vi "SS2 Live_Next Image Acquisition Step.vi"(8 "Error In":errorcluster, 9 "Message in":string, 11 "SS2 Live Internal Variables in":T3={"okCFrontPanelDevices Refnum"=refnum, "Device Refnum"=refnum, "Display Image"=refnum, "# Live Images"=0, "relative s"=0.0, "# Image Sets"=0, "Message"="", "Current Image Set"=0, "# Datasets"=0, "Current Dataset"=0, "Live Mode"=FALSE, "Recording Mode"=FALSE, "Record Button"=refnum, "Live Button"=refnum, "SS2 Live Gate Data Q Name"="SS2 Live Gate Data Q", "Discard First Image"=FALSE, "Image Information"={"Save ROI Only"=FALSE, "Left"=0, "Top"=0, "Right"=0, "Bottom"=0, "Use Current ROI"=FALSE}, "Image Binning Options"={"Use Image Binning"=FALSE, "X Bin"=1, "Y Bin"=1}} {"Image Binning Options"."Y Bin" min=1; "Image Binning Options"."X Bin" min=1}) -> (0 "Error Out":errorcluster, 1 "Message out":string, 2 "SS2 Live Atomic Action":T1={"SS2 Q Event"=enum."Idle", "Data"=variant}, 3 "SS2 Live Internal Variables out":T3={"okCFrontPanelDevices Refnum"=refnum, "Device Refnum"=refnum, "Display Image"=refnum, "# Live Images"=0, "relative s"=0.0, "# Image Sets"=0, "Message"="", "Current Image Set"=0, "# Datasets"=0, "Current Dataset"=0, "Live Mode"=FALSE, "Recording Mode"=FALSE, "Record Button"=refnum, "Live Button"=refnum, "SS2 Live Gate Data Q Name"="SS2 Live Gate Data Q", "Discard First Image"=FALSE, "Image Information"={"Save ROI Only"=FALSE, "Left"=0, "Top"=0, "Right"=0, "Bottom"=0, "Use Current ROI"=FALSE}, "Image Binning Options"={"Use Image Binning"=FALSE, "X Bin"=1, "Y Bin"=1}} {"Image Binning Options"."Y Bin" min=1; "Image Binning Options"."X Bin" min=1})   [LabVIEW 2019]
uses:
  SS2 Live Internal Variables.ctl
  C:/UCLA Thinkpad Google Drive/LabVIEW 2019 SP1/builds/SS2 Live Distribution/Opal Kelly/C# Wrapper/libFrontPanel-csharp.dll
  Opal Kelly/C# Wrapper/libFrontPanel-csharp.dll
  <vilib>/vision/Image Controls.llb/IMAQ Image.ctl
  SS2 Live_Image ROI Information.ctl
  Phasor/Image Binning Options.ctl
  SS2 Q [Element].ctl
  SS2 Q Event List.ctl
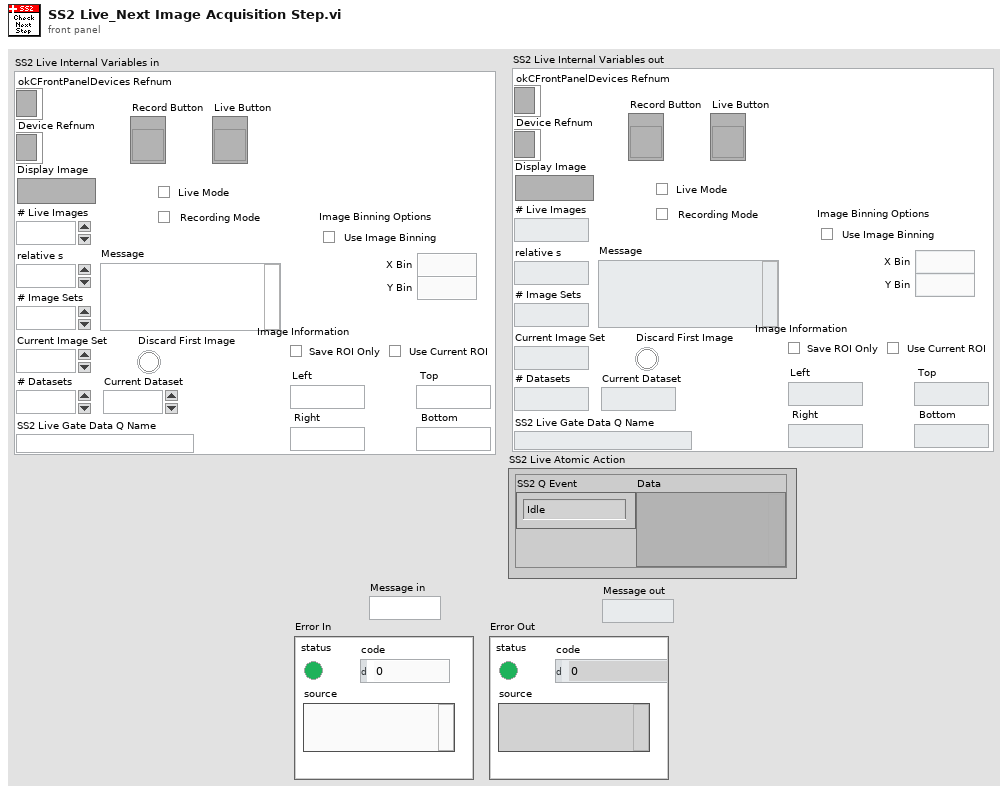
[diagram p1: front panel]
types:
  T1 = typedef "SS2 Q [Element].ctl" = cluster{"SS2 Q Event":T2, "Data":variant}
  T2 = typedef "SS2 Q Event List.ctl" = enum16{"---- UI ----", "Idle", "Initialization", "Quit", "---- DAQ ----", "Start Recording", "Start Live Acquisition", "Initialize Recording Mode", "Initialize FPGA (Live Mode)", "Get Image Set", "Get Single Image", "Update Image Display", "Stop Live Acquisition", "Stop Data Recording", "---- Image ----", "Copy Data to Clipboard", "Set Image Palette", "Save Displayed Image with Overlay", "Save Image Data as TIFF"}
  T3 = typedef "SS2 Live Internal Variables.ctl" = cluster{"okCFrontPanelDevices Refnum":refnum<k24>, "Device Refnum":refnum<k24>, "Display Image":T4, "# Live Images":i32, "relative s":dbl, "# Image Sets":i32, "Message":string, "Current Image Set":i32, "# Datasets":i32, "Current Dataset":i32, "Live Mode":bool, "Recording Mode":bool, "Record Button":refnum<vi>, "Live Button":refnum<vi>, "SS2 Live Gate Data Q Name":string, "Discard First Image":bool, "Image Information":T5, "Image Binning Options":T6}
  T4 = typedef "IMAQ Image.ctl" = refnum<image>
  T5 = typedef "SS2 Live_Image ROI Information.ctl" = cluster{"Save ROI Only":bool, "Left":u16, "Top":u16, "Right":u16, "Bottom":u16, "Use Current ROI":bool}
  T6 = typedef "Image Binning Options.ctl" = cluster{"Use Image Binning":bool, "X Bin":i32, "Y Bin":i32}
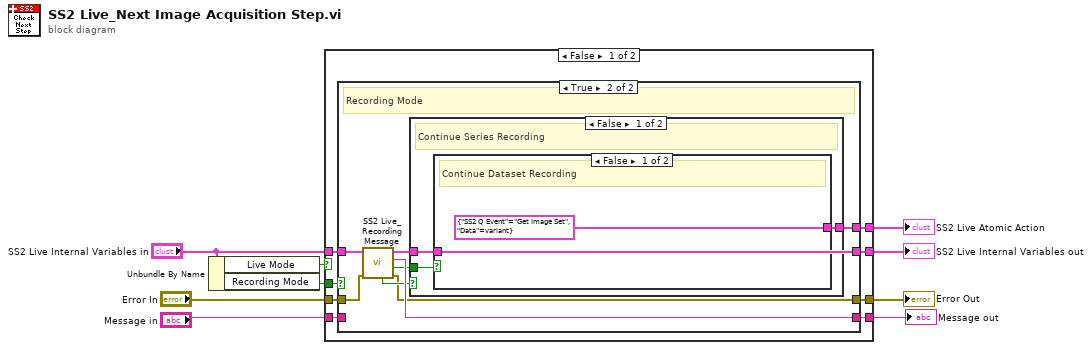
[diagram p0: block diagram]
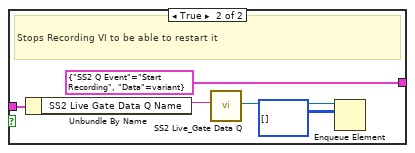
[diagram p3: hidden frame]
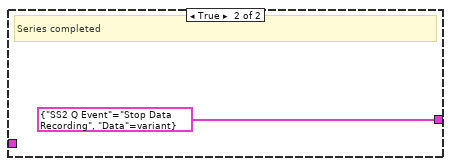
[diagram p4: hidden frame]
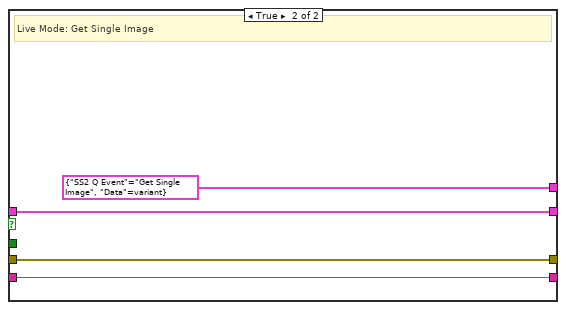
[diagram p5: hidden frame]
diagram:
  n1 = Unbundle By Name("SS2 Live Internal Variables in") -> ("Live Mode"=w5:bool, "Recording Mode"=w7:bool)
  n2 = case shown="False" w5 {
    tunnel: [w12 T1 {"SS2 Q Event"=enum."Get Single Image", "Data"=variant} ("SS2 Live Atomic Action")] -> w6
    tunnel: w7 -> [w13 _]
    tunnel: "SS2 Live Internal Variables in" -> [w17 w41]
    tunnel: [w16 w41] -> w9
    tunnel: "Error In" -> [w15 w40]
    tunnel: [w11 w40] -> w3
    tunnel: [w14 w39] -> w2
    tunnel: "Message in" -> [w10 w39]
    frame False {
      n3 = case shown="True" w13 {
        tunnel: w17 -> [w20 w28]
        tunnel: [w20 w21] -> w16
        tunnel: w15 -> [w19 w27]
        tunnel: [w18 w26] -> w14
        tunnel: [_ w24] -> w12
        tunnel: [w19 w22] -> w11
        tunnel: w10 -> [w18 _]
        frame False {
          # "Nop"
        }
        frame True {
          # "Recording Mode"
          n4 = call "SS2 Live_Recording Message.vi"("error in (no error)"=w27, "SS2 Live Internal Variables"=w28) -> ("error out"=w22:errorcluster, "Current Dataset Recording Completed?"=w23:bool, "Message"=w26:string, "SS2 Live Internal Variables"=w21:T3, "Dataset Series Completed?"=w25:bool)  [unwired: 5 in]
          n5 = case shown="False" w25 {
            tunnel: [w31 T1 {"SS2 Q Event"=enum."Stop Data Recording", "Data"=variant} ("SS2 Live Atomic Action")] -> w24
            tunnel: w23 -> [w30 _]
            tunnel: w21 -> [w29 _]
            frame False {
              # "Continue Series Recording"
              n6 = case shown="False" w30 {
                tunnel: [T1 {"SS2 Q Event"=enum."Get Image Set", "Data"=variant} ("SS2 Live Atomic Action") T1 {"SS2 Q Event"=enum."Start Recording", "Data"=variant} ("SS2 Live Atomic Action")] -> w31
                tunnel: w29 -> [_ w35]
                frame False {
                  # "Continue Dataset Recording"
                }
                frame True {
                  # "Stops Recording VI to be able to restart it"
                  n7 = Unbundle By Name(w35) -> ("SS2 Live Gate Data Q Name"=w34:string)
                  n8 = call "SS2 Live_Gate Data Q.vi"("SS2 Live Gate Data Q Name"=w34) -> ("SS2 Live Gate Data Q"=w37:refnum<queue>)  [unwired: 5 in, 1 out]
                  n9 = Enqueue Element(queue=w37, element=u8[][] []) -> ()  [unwired: 2 in, 3 out]
                }
              }
            }
            frame True {
              # "Series completed"
            }
          }
        }
      }
    }
    frame True {
      # "Live Mode: Get Single Image"
    }
  }
  "SS2 Live Internal Variables out" <- w9
  "SS2 Live Atomic Action" <- w6
  "Error Out" <- w3
  "Message out" <- w2
